vi "Build List of Items for Tree.vi"(8 "error in (no error)":errorcluster, 11 "output cluster":T2) -> (0 "error out":errorcluster, 2 "FileTree":T1(array[cluster]), 3 "TreeItems":T1(array[cluster]))   [LabVIEW 2018]
doc: "Convert cluster containing Groups, Channels (datasets and sub datasets), and file paths into nested tree items that can be appended to Tree."
uses:
  ItemsInFile_Clust.ctl
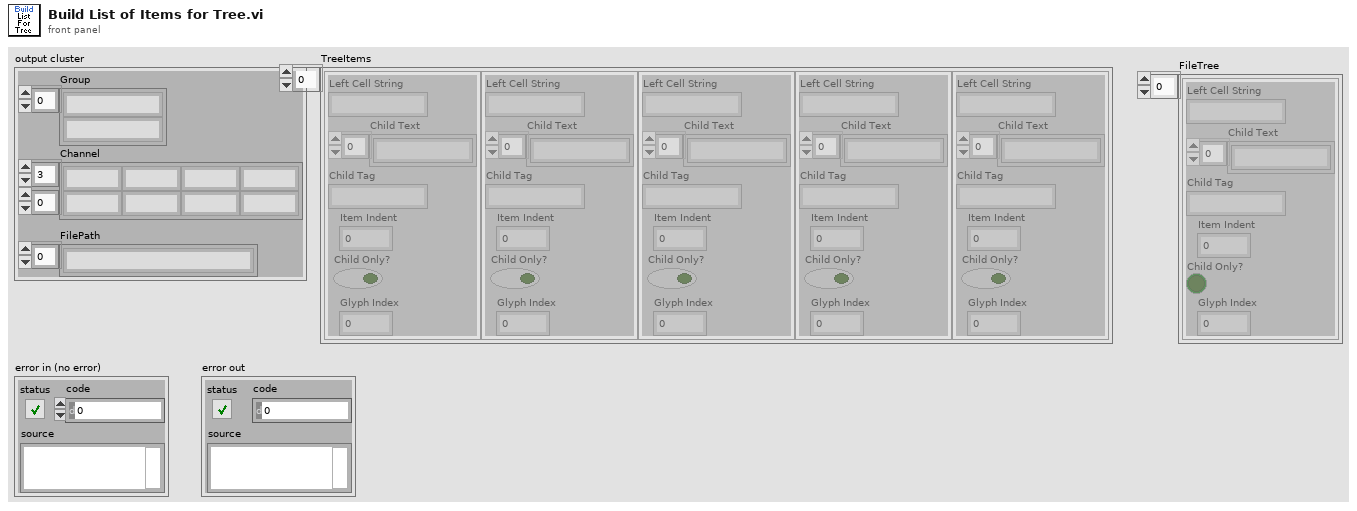
[diagram p1: front panel]
types:
  T1 = cluster{"Left Cell String":string, "Child Text":string[], "Child Tag":string, "Item Indent":i32, "Child Only?":bool, "Glyph Index":i32}[]
  T2 = typedef "ItemsInFile_Clust.ctl" = cluster{"Group":string[], "Channel":string[][], "FilePath":string[]}
  T3 = cluster{"Left Cell String":string, "Child Text":string[], "Child Tag":string, "Item Indent":i32, "Child Only?":bool, "Glyph Index":i32}
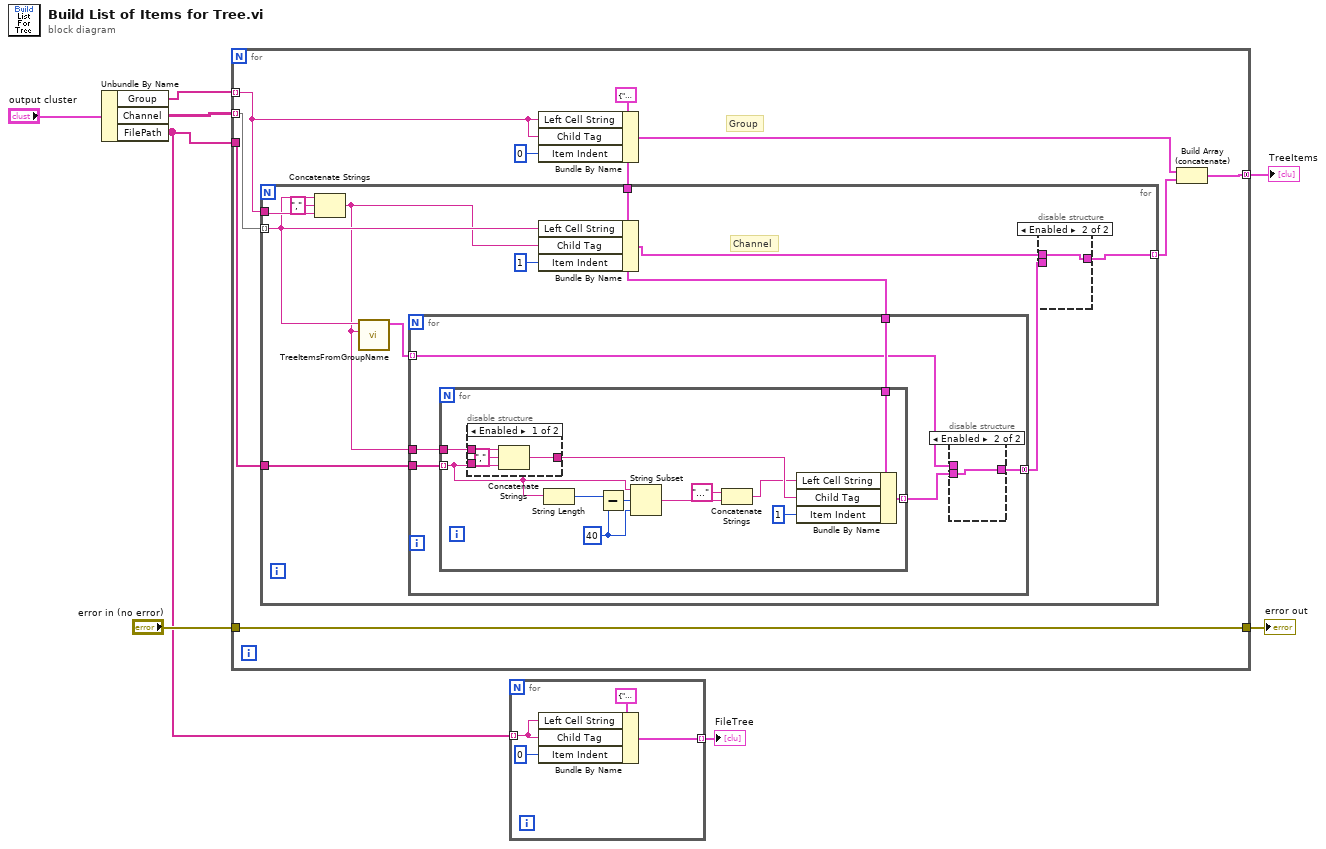
[diagram p0: block diagram]
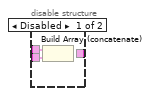
[diagram p2: hidden frame]
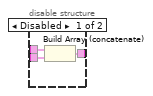
[diagram p3: hidden frame]
diagram:
  n1 = Unbundle By Name("output cluster") -> ("Group"=w6:string[], "Channel"=w7:string[][], "FilePath"=w2:string[])
  n2 = for {
    tunnel: "error in (no error)" -> [w16]
    tunnel: w6 -> [w10] mode=indexing
    tunnel: w7 -> [w15] mode=indexing
    tunnel: [w12] -> w4 mode=concatenating
    tunnel: [w16] -> w3
    tunnel: w2 -> [w9]
    w11 = T3 {"Left Cell String"="", "Child Text"=[], "Child Tag"="", "Item Indent"=0, "Child Only?"=FALSE, "Glyph Index"=0} ("Item")
    # "Group"
    n3 = for {
      tunnel: w15 -> [w19] mode=indexing
      tunnel: [w23] -> w14 mode=indexing
      tunnel: w11 -> [w24]
      tunnel: w10 -> [w27]
      tunnel: w9 -> [w25]
      # "Channel"
      n4 = Concatenate Strings(w19, "," ("string"), w27) -> (w18:string)
      n5 = call "TreeItemsFromGroupName.vi"("Child Tag"=w18, "String"=w19) -> ("ClusterItemTreeEntries"=w21:T1)  [unwired: 7 in, 2 out]
      n6 = for {
        tunnel: w25 -> [w37]
        tunnel: w24 -> [w36]
        tunnel: w18 -> [w32]
        tunnel: w21 -> [w35] mode=indexing
        tunnel: [w33] -> w20 mode=concatenating
        n7 = for {
          tunnel: w37 -> [w44] mode=indexing
          tunnel: w32 -> [w52]
          tunnel: w36 -> [w51]
          tunnel: [w50] -> w34 mode=indexing
          w48 = 40
          n8 = disable-structure shown="Enabled" {
            disable-tunnel: w52 -> [w56 _]
            disable-tunnel: [w55 w58] -> w49
            disable-tunnel: w44 -> [w54 w58]
            frame Enabled {
              n9 = Concatenate Strings(w56, "," ("string"), w54) -> (w55:string)
            }
            frame Disabled {
            }
          }
          n10 = String Length(string=w44) -> (length=w46:i32)
          n11 = Subtract(x=w46, y=w48) -> (x-y=w47:i32)
          n12 = String Subset(string=w44, offset (0)=w47, length (rest)=w48) -> (substring=w45:string)
          n13 = Concatenate Strings("..." ("string"), w45) -> (w43:string)
          n14 = Bundle By Name(cluster=w51, "Left Cell String"=w43, "Child Tag"=w49, "Item Indent"=1) -> (w50:T3)
        }
        n15 = disable-structure shown="Enabled" {
          disable-tunnel: w35 -> [w40 _]
          disable-tunnel: w34 -> [w39 w41]
          disable-tunnel: [w38 w41] -> w33
          frame Disabled {
            n16 = Build Array (concatenate)(w40, w39) -> (w38:T1)
          }
          frame Enabled {
          }
        }
      }
      n17 = Bundle By Name(cluster=w24, "Left Cell String"=w19, "Child Tag"=w18, "Item Indent"=1) -> (w22:T3)
      n18 = disable-structure shown="Enabled" {
        disable-tunnel: [_ w31] -> w23
        disable-tunnel: w22 -> [w30 w31]
        disable-tunnel: w20 -> [w29 _]
        frame Disabled {
          n19 = Build Array (concatenate)(w30, w29) -> ()  [unwired: 1 out]
        }
        frame Enabled {
        }
      }
    }
    n20 = Bundle By Name(cluster=w11, "Left Cell String"=w10, "Child Tag"=w10, "Item Indent"=0) -> (w13:T3)
    n21 = Build Array (concatenate)(w13, w14) -> (w12:T1)
  }
  "TreeItems" <- w4
  "error out" <- w3
  n22 = for {
    tunnel: w2 -> [w60] mode=indexing
    tunnel: [w59] -> w1 mode=indexing
    n23 = Bundle By Name(cluster=T3 {"Left Cell String"="", "Child Text"=[], "Child Tag"="", "Item Indent"=0, "Child Only?"=FALSE, "Glyph Index"=0} ("Item"), "Left Cell String"=w60, "Child Tag"=w60, "Item Indent"=0) -> (w59:T3)
  }
  "FileTree" <- w1
